vi "9610 Missing mandatory sub-index--error.vi"(8 "error in":errorcluster, 10 "Sub-Index":u16, 11 "Index":u16) -> (0 "error out":errorcluster)   [LabVIEW 2019, in "Electronic Datasheet.lvlib"]
uses:
  Electronic Datasheet.lvlib
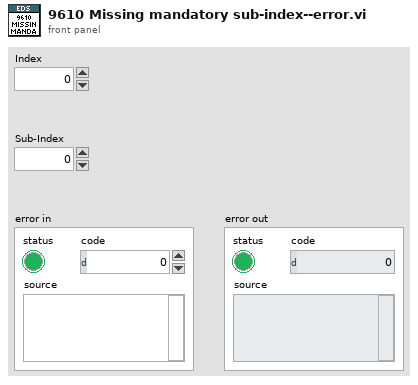
[diagram p1: front panel]
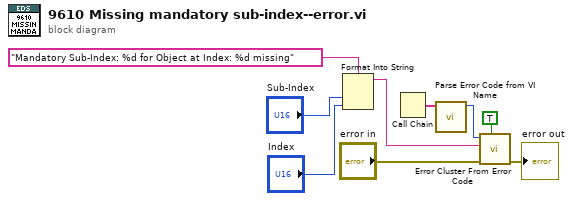
[diagram p0: block diagram]
diagram:
  n1 = Format Into String(format string="Mandatory Sub-Index: %d for Object at Index: %d missing", "Sub-Index", "Index") -> (resulting string=w6:string)  [unwired: 2 in, 1 out]
  n2 = Call Chain() -> (call chain=w1:string[])
  n3 = call "Parse Error Code from VI Name.vi"("Call Chain"=w1) -> ("Error Code"=w2:i32)  [unwired: 10 in]
  n4 = call <vilib>:"Error Cluster From Error Code.vi"("show call chain? (False)"=TRUE, "error in (no error)"="error in", "error message (\"\")"=w6, "error code (0)"=w2) -> ("error out"=→"error out":errorcluster)  [unwired: 5 in]
